vi "Read DecPlace.vi"(8 "error in":errorcluster, 11 "CN79000 in":refnum<class "CN79000.lvclass">=refnum) -> (0 "error out":errorcluster, 2 "DecPt":i32[](array[numeric]), 3 "CN79000 out":refnum<class "CN79000.lvclass">)   [LabVIEW 2014, in "CN79000.lvclass"]
uses:
  CN79000.lvclass
  Build Command-Single Val.vi
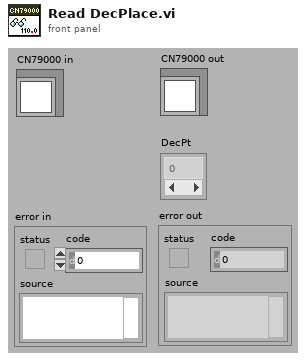
[diagram p1: front panel]
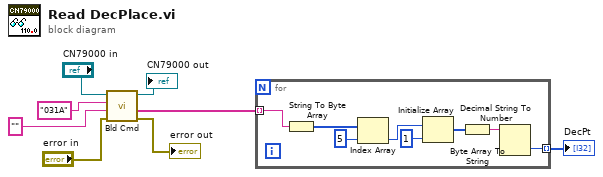
[diagram p0: block diagram]
diagram:
  n1 = call-poly "Bld Cmd.vi"("error in"="error in", "Val"="" ("Cmd"), "Cmd"="031A" ("string"), "CN79000 in"="CN79000 in") -> ("error out"=→"error out":errorcluster, "DataOut"=w3:string[], "CN79000 out"=→"CN79000 out":refnum<class "CN79000.lvclass">)  [unwired: 3 in, 1 out]
  n2 = for {
    tunnel: [w10] -> w8 mode=indexing
    tunnel: w3 -> [w9] mode=indexing
    n3 = String To Byte Array(string=w9) -> (unsigned byte array=w11:u8[])
    n4 = Index Array(array=w11, index=5) -> (element=w13:u8)
    n5 = Initialize Array(w13, 1 ("dimension size")) -> (w15:u8[])
    n6 = Byte Array To String(unsigned byte array=w15) -> (string=w16:string)
    n7 = Decimal String To Number(string=w16) -> (number=w10:i32)  [unwired: 2 in, 1 out]
  }
  "DecPt" <- w8
